vi "Teleop.vi"(10 "Match Info":T1={"Autonomous Elapsed Seconds"=0.0, "TeleOp Elapsed Seconds"=0.0, "Disabled Elapsed Seconds"=0.0, "Visited Autonomous"=FALSE, "Visited TeleOp"=FALSE, "Visited Disabled"=FALSE, "Autonomous Settings"={"Autonomous Style"=enum."Independent", "VI Refnum"=refnum}}, 11 "Call Context":T2) -> ()   [LabVIEW 2014]
doc: "This VI is called for each TeleOp packet received from the DS where the robot is not disabled. It is often used to read from the joysticks and update I/O or to update setpoints for timed control loops. It should complete and return within 20 milliseconds or it may miss DS packets."
uses:
  <vilib>/Rock Robotics/WPI/DriverStation/WPI_DriverStationDerivedRobotMode.ctl
  <vilib>/Rock Robotics/WPI/DriverStation/WPI_DriverStationMatch Info.ctl
  <vilib>/Rock Robotics/WPI/Ultrasonic/WPI_UltrasonicRangeUnits.ctl
  <vilib>/Rock Robotics/WPI/Joystick/WPI_JoystickGetSetRefNum.vi
  <vilib>/Rock Robotics/Network Tables/SD Write Boolean Array.vi
  <vilib>/Rock Robotics/Network Tables/SD Write Numeric Array.vi
  <vilib>/Rock Robotics/Network Tables/SD Read Boolean.vi
  <vilib>/Rock Robotics/Network Tables/SD Read Number.vi
  <vilib>/Rock Robotics/WPI/Ultrasonic/WPI_SonarSRF04DigitalRefNum Registry Get.vi
  <vilib>/Rock Robotics/WPI/Ultrasonic/WPI_SonarSRF04DigitalGetRange.vi
panel:
  in  "Angle":i32
  out "Distance":dbl
  out "Rotation Angle":u16
  out "Camera Angle":u16
  out "x 2":dbl
  out "y 2":dbl
  out "y":dbl
  out "x":dbl
  out "Sample Slider 0":dbl(slide) scale=0.0..5.0
  out "Sample Boolean 1":bool
  out "Sample Boolean 0":bool
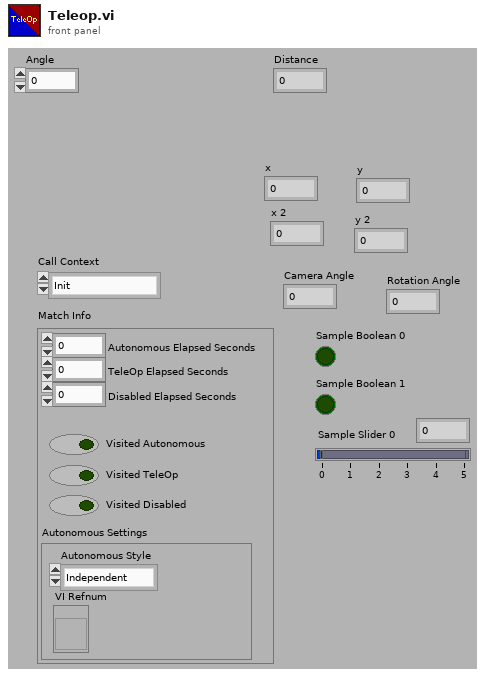
[diagram p1: front panel]
types:
  T1 = typedef "WPI_DriverStationMatch Info.ctl" = cluster{"Autonomous Elapsed Seconds":dbl, "TeleOp Elapsed Seconds":dbl, "Disabled Elapsed Seconds":dbl, "Visited Autonomous":bool, "Visited TeleOp":bool, "Visited Disabled":bool, "Autonomous Settings":cluster{"Autonomous Style":enum16{"Iterative", "Independent"}, "VI Refnum":refnum<vi>}}
  T2 = typedef "WPI_DriverStationDerivedRobotMode.ctl" = enum16{"Init", "Execute", "Stop"}
  T3 = typedef "WPI_UltrasonicRangeUnits.ctl" = enum16{"inches", "mm"}
  T4 = typedef "WPI_JoystickDevRef.ctl" = cluster{"Device":T5}
  T5 = typedef "WPI_JoystickDeviceEnum.ctl" = enum16{"USB 0", "USB 1", "USB 2", "USB 3", "USB 4", "USB 5"}
  T6 = typedef "WPI_ServoDeviceRef.ctl" = cluster{"DeviceStatus":errorcluster, "Controller":T7, "PWM Channel":T8, "DeadBand":T9}
  T7 = typedef "FPGA_TypedefDigitalModule.ctl" = enum16{"Controller 1"}
  T8 = typedef "FPGA_DIOPWMChannel.ctl" = enum8{"PWM 0", "PWM 1", "PWM 2", "PWM 3", "PWM 4", "PWM 5", "PWM 6", "PWM 7", "PWM 8", "PWM 9", "PWM MXP 0", "PWM MXP 1", "PWM MXP 2", "PWM MXP 3", "PWM MXP 4", "PWM MXP 5", "PWM MXP 6", "PWM MXP 7", "PWM MXP 8", "PWM MXP 9", "Invalid"}
  T9 = typedef "WPI_PWMDeadband.ctl" = cluster{"Name":string, "maxPositivePwm":i32, "minPositivePwm":i32, "centerPwm":i32, "maxNegativePwm":i32, "minNegativePwm":i32, "angularRange":u16}
  T10 = typedef "WPI_UltrasonicDeviceRef.ctl" = cluster{"DevStatus":errorcluster, "Ping Digital Controller":T7, "Echo Digital Controller":T7, "Ping Channel":T11, "Echo Channel":T11, "CntIndex":T12}
  T11 = typedef "FPGA_DIOChannel.ctl" = enum8{"DIO 0", "DIO 1", "DIO 2", "DIO 3", "DIO 4", "DIO 5", "DIO 6", "DIO 7", "DIO 8", "DIO 9", "DIO MXP 0", "DIO MXP 1", "DIO MXP 2", "DIO MXP 3", "DIO MXP 4", "DIO MXP 5", "DIO MXP 6", "DIO MXP 7", "DIO MXP 8", "DIO MXP 9", "DIO MXP 10", "DIO MXP 11", "DIO MXP 12", "DIO MXP 13", "DIO MXP 14", "DIO MXP 15", "Invalid"}
  T12 = typedef "FPGA_CounterCtrSystemIndex.ctl" = enum8{"Ctr 0", "Ctr 1", "Ctr 2", "Ctr 3", "Ctr 4", "Ctr 5", "Ctr 6", "Ctr 7", "Invalid"}
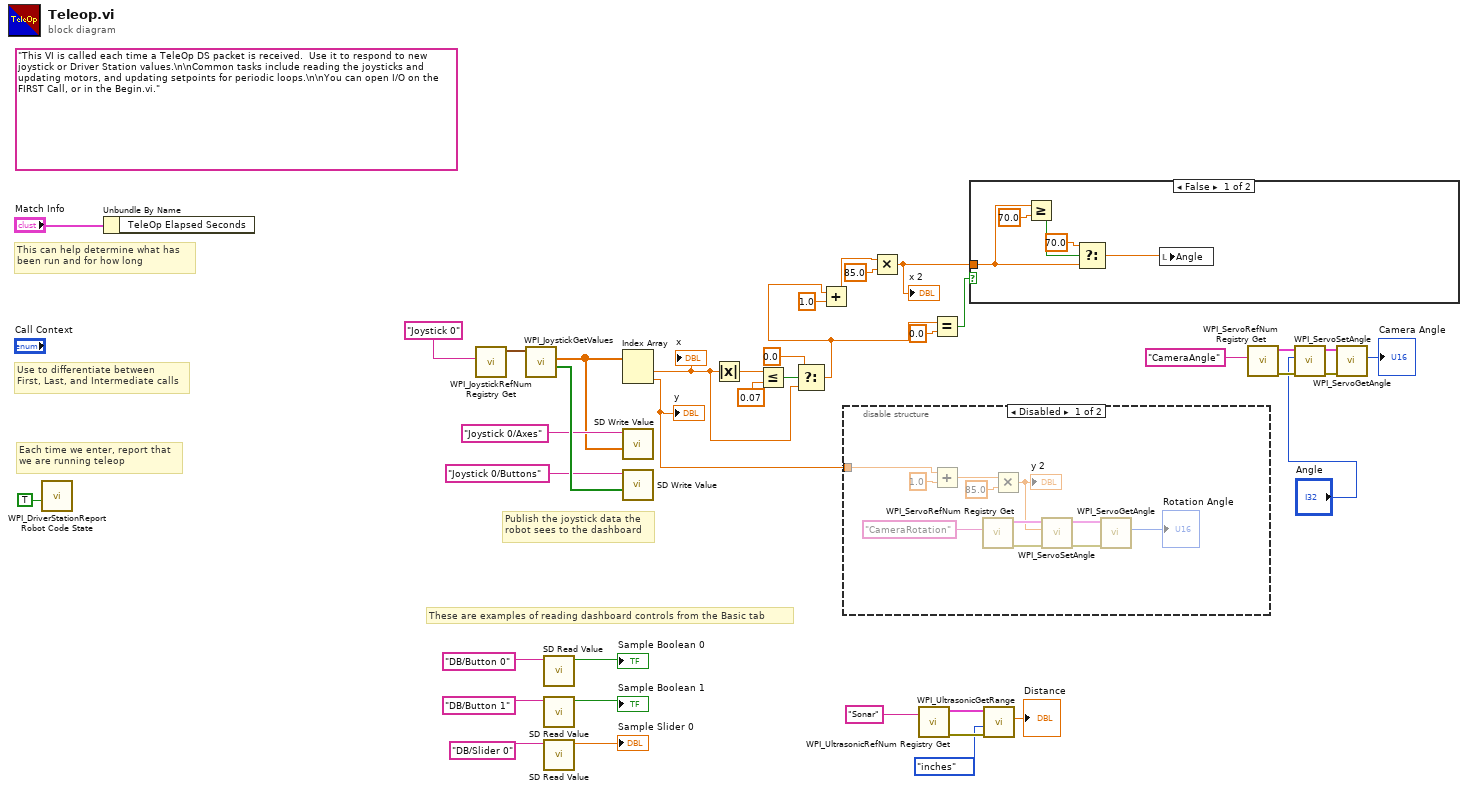
[diagram p0: block diagram]
diagram:
  (unwired) "This VI is called each time a TeleOp DS packet is received.  Use it to respond to new joystick or Driver Station values.\n\nCommon tasks include reading the joysticks and updating motors, and updating setpoints for periodic loops.\n\nYou can open I/O on the FIRST Call, or in the Begin.vi."
  # "These are examples of reading dashboard controls from the Basic tab"
  # "Publish the joystick data the\nrobot sees to the dashboard"
  # "Each time we enter, report that\nwe are running teleop"
  # "Use to differentiate between\nFirst, Last, and Intermediate calls"
  # "This can help determine what has\nbeen run and for how long"
  n1 = call <vilib>:"WPI_DriverStationReport Robot Code State.vi"("TeleOp"=TRUE ("Autonomous")) -> ()  [unwired: 10 in, 1 out]
  n2 = Unbundle By Name("Match Info") -> ()  [unwired: 1 out]
  n3 = call <vilib>:"WPI_JoystickRefNum Registry Get.vi"("refnum name"="Joystick 0") -> ("JoystickDevRef"=w37:T4)  [unwired: 1 in, 9 out]
  n4 = call <vilib>:"WPI_JoystickGetValues.vi"("JoystickDevRef"=w37) -> ("Buttons"=w35:bool[], "Axes"=w26:dbl[])  [unwired: 6 in, 3 out]
  n5 = call-poly <vilib>:"SD Read Value.vi"("Name"="DB/Button 0" ("refnum name")) -> ("Boolean"=→"Sample Boolean 0":bool)  [unwired: 8 in, 2 out]
  n6 = call-poly <vilib>:"SD Read Value.vi"("Name"="DB/Button 1" ("refnum name")) -> ("Boolean"=→"Sample Boolean 1":bool)  [unwired: 8 in, 2 out]
  n7 = call-poly <vilib>:"SD Read Value.vi"("Name"="DB/Slider 0" ("refnum name")) -> ("Numeric"=→"Sample Slider 0":dbl)  [unwired: 8 in, 2 out]
  n8 = Index Array(array=w26) -> (element #1=w16:dbl, element #2=w24:dbl)  [unwired: 2 in]
  "x" <- w16
  "y" <- w24
  n9 = call-poly <vilib>:"SD Write Value.vi"("Numeric Array"=w26, "Name"="Joystick 0/Axes") -> ()  [unwired: 8 in, 2 out]
  n10 = call-poly <vilib>:"SD Write Value.vi"("Boolean Array"=w35, "Name"="Joystick 0/Buttons") -> ()  [unwired: 8 in, 2 out]
  n11 = Absolute Value(x=w16) -> (abs(x)=w17:dbl)
  n12 = Less Or Equal?(x=w17, y=0.07) -> (x <= y?=w19:bool)
  n13 = Select(t=0.0, s=w19, f=w16) -> (s? t:f=w13:dbl)
  n14 = Add(x=w13, y=1.0) -> (x+y=w14:dbl)
  n15 = disable-structure shown="Disabled" {
    disable-tunnel: w24 -> [w47 _]
    frame Disabled {
      n16 = Add(x=w47, y=1.0) -> (x+y=w49:dbl)
      n17 = call <vilib>:"WPI_ServoRefNum Registry Get.vi"("refnum name"="CameraRotation") -> ("error out"=w43:errorcluster, "ServoDeviceRef"=w44:T6)  [unwired: 9 in]
      n18 = Multiply(x=w49, y=85.0) -> (x*y=w40:dbl)
      "y 2" <- w40
      n19 = call <vilib>:"WPI_ServoSetAngle.vi"("error in (no error)"=w43, "Angle"=w40, "ServoDeviceRef"=w44) -> ("error out"=w41:errorcluster, "ServoDeviceRef"=w42:T6)  [unwired: 7 in]
      n20 = call <vilib>:"WPI_ServoGetAngle.vi"("ServoDeviceRef"=w42, "error in (no error)"=w41) -> ("Angle"=→"Rotation Angle":u16)  [unwired: 6 in, 2 out]
    }
    frame Enabled {
    }
  }
  n21 = Multiply(x=w14, y=85.0) -> (x*y=w21:dbl)
  "x 2" <- w21
  n22 = call-poly <vilib>:"WPI_UltrasonicRefNum Registry Get.vi"("refnum name"="Sonar") -> ("error out"=w11:errorcluster, "SonarSRF04DevRef"=w12:T10)  [unwired: 9 in]
  n23 = Equal?(x=w13, y=0.0) -> (x = y?=w23:bool)
  n24 = case shown="False" w23 {
    tunnel: w21 -> [w52 _]
    frame False {
      n25 = Greater Or Equal?(x=w52, y=70.0) -> (x >= y?=w54:bool)
      n26 = Select(t=70.0 ("y"), s=w54, f=w52) -> (s? t:f=w51:dbl)
      n27 = local write "Angle"(w51) -> ()
    }
    frame True {
    }
  }
  n28 = call-poly <vilib>:"WPI_UltrasonicGetRange.vi"("error in (no error)"=w11, "Range Units"=WPI_UltrasonicRangeUnits."inches", "SonarSRF04DevRef"=w12) -> ("Distance"=→"Distance":dbl)  [unwired: 6 in, 2 out]
  n29 = call <vilib>:"WPI_ServoRefNum Registry Get.vi"("refnum name"="CameraAngle") -> ("error out"=w2:errorcluster, "ServoDeviceRef"=w5:T6)  [unwired: 9 in]
  n30 = call <vilib>:"WPI_ServoSetAngle.vi"("error in (no error)"=w2, "Angle"="Angle", "ServoDeviceRef"=w5) -> ("error out"=w3:errorcluster, "ServoDeviceRef"=w4:T6)  [unwired: 7 in]
  n31 = call <vilib>:"WPI_ServoGetAngle.vi"("ServoDeviceRef"=w4, "error in (no error)"=w3) -> ("Angle"=→"Camera Angle":u16)  [unwired: 6 in, 2 out]
